vi "Close.vi"(8 "error in (no error)":errorcluster, 11 "BT in":refnum<class "BT.lvclass">) -> (0 "error out":errorcluster, 3 "BT out":refnum<class "BT.lvclass">)   [LabVIEW 2014, in "BT.lvlib" / "BT.lvclass"]
uses:
  BT.lvclass
  BT.lvclass/BT.ctl
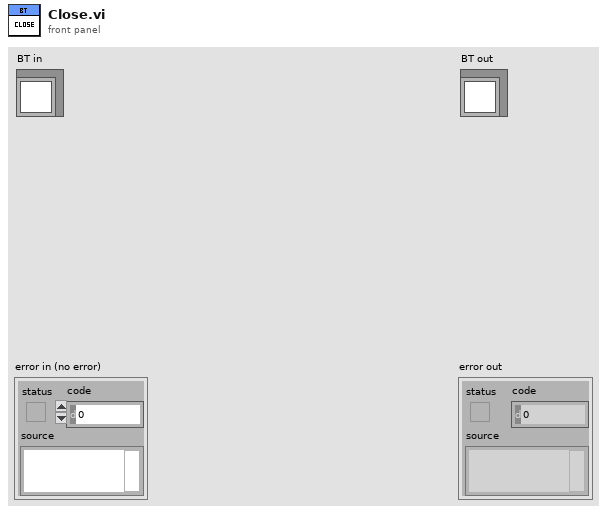
[diagram p1: front panel]
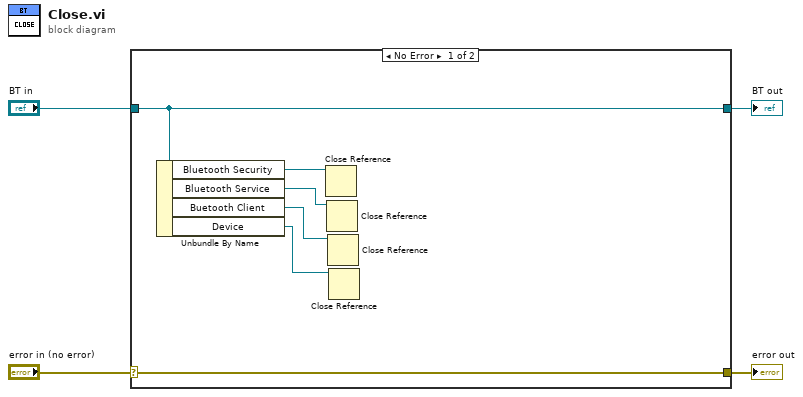
[diagram p0: block diagram]
diagram:
  n1 = case shown="No Error" "error in (no error)" {
    selector: "error in (no error)" -> [w10 w12]
    tunnel: [w10 w12] -> w3
    tunnel: [w9 w11] -> w1
    tunnel: "BT in" -> [w9 w11]
    frame No Error {
      n2 = Unbundle By Name(w9) -> ("Bluetooth Security"=w8:refnum<k24>, "Bluetooth Service"=w7:refnum<k24>, "Buetooth Client"=w6:refnum<k24>, "Device"=w5:refnum<k24>)
      n3 = Close Reference(reference=w8) -> ()  [unwired: 1 in, 1 out]
      n4 = Close Reference(reference=w7) -> ()  [unwired: 1 in, 1 out]
      n5 = Close Reference(reference=w6) -> ()  [unwired: 1 in, 1 out]
      n6 = Close Reference(reference=w5) -> ()  [unwired: 1 in, 1 out]
    }
    frame Error {
    }
  }
  "error out" <- w3
  "BT out" <- w1
